vi "Create New Bucket.vi"() -> ()   [LabVIEW 2015]
doc: "Demonstrates the use of the <b>Create Bucket</b> VI in the LabVIEW Interface for Amazon S3 toolkit."
uses:
  Typedefs/AMZ_S3_LocationConstraint.ctl
  Typedefs/AMZ_S3_AWS Credentials.ctl
  Typedefs/AMZ_S3_API_PUT Bucket Request Parameters.ctl
  Typedefs/AMZ_S3_ACL.ctl
  LV Interface for Amazon S3.lvlib
panel:
  in  "Secret Key":string
  in  "Access Key":string
  in  "Bucket Name":string
  in  "Region":T1
  # "Overview: Demonstrates how to create a new Amazon S3 bucket.\nRequirements: LabVIEW Interface for Amazon S3 toolkit and a registered Amazon AWS account\nInstructions:\n1. Specify the Access Key and Secret Key for your AWS account. You can create an account at http://aws.amazon.com.\n2. Specify a Region and Bucket Name for the bucket you want to create. Note that the bucket name must be globally unique.\n3. Run the VI. Verify in the Amazon S3 console that the specified bucket was created."
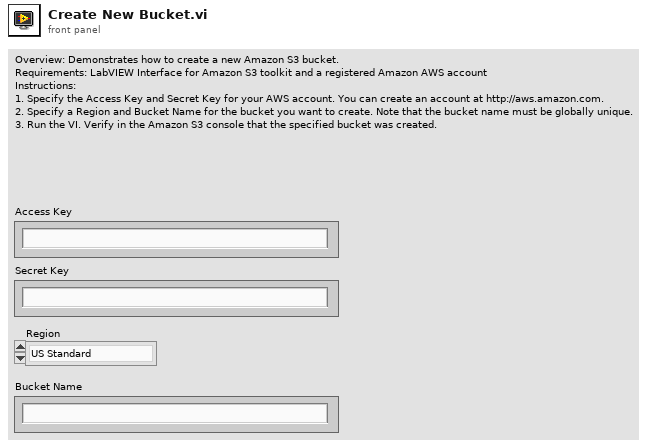
[diagram p1: front panel]
types:
  T1 = typedef "LV Interface for Amazon S3.lvlib/AMZ_S3_LocationConstraint.ctl" = enum16{"US Standard", "us-east-2", "us-west-1", "us-west-2", "ap-northeast-1", "ap-northeast-2", "ap-southeast-1", "ap-southeast-2", "ca-central-1", "eu-central-1", "eu-west-1", "eu-west-2", "sa-east-1"}
  T2 = typedef "LV Interface for Amazon S3.lvlib/AMZ_S3_AWS Credentials.ctl" = cluster{"Access Key":string, "Secret Key":string}
  T3 = typedef "LV Interface for Amazon S3.lvlib/AMZ_S3_API_PUT Bucket Request Parameters.ctl" = cluster{"ACL":T4, "Region":T1}
  T4 = typedef "LV Interface for Amazon S3.lvlib/AMZ_S3_ACL.ctl" = enum16{"private", "public-read", "public-read-write", "aws-exec-read", "authenticated-read", "bucket-owner-read", "bucket-owner-full-control"}
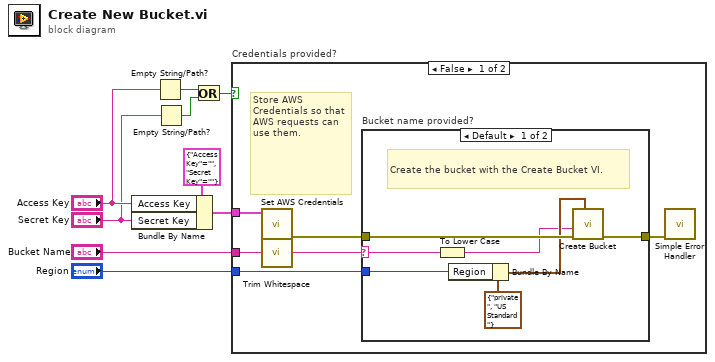
[diagram p0: block diagram]
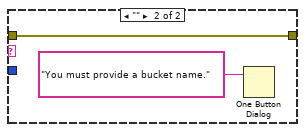
[diagram p2: hidden frame]
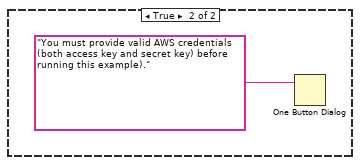
[diagram p3: hidden frame]
diagram:
  n1 = Bundle By Name(cluster=T2 {"Access Key"="", "Secret Key"=""} ("AWS Credentials in"), "Access Key"="Access Key", "Secret Key"="Secret Key") -> (w8:T2)
  n2 = Empty String/Path?(string/path="Access Key") -> (empty?=w7:bool)
  n3 = Empty String/Path?(string/path="Secret Key") -> (empty?=w5:bool)
  n4 = Or(x=w7, y=w5) -> (x .or. y?=w6:bool)
  n5 = case "Credentials provided?" shown="False" w6 {
    tunnel: w8 -> [w15 _]
    tunnel: "Bucket Name" -> [w12 _]
    tunnel: "Region" -> [w10 _]
    frame False {
      # "Store AWS Credentials so that AWS requests can use them."
      n6 = call "Set AWS Credentials.vi"("AWS Credentials in"=w15) -> ("error out"=w14:errorcluster)  [unwired: 10 in]
      n7 = call <vilib>:"Trim Whitespace.vi"("string"=w12) -> ("trimmed string"=w11:string)  [unwired: 1 in]
      n8 = case "Bucket name provided?" shown="Default" w11 {
        selector: w11 -> [w20 _]
        tunnel: w14 -> [w21 w24]
        tunnel: [w18 w24] -> w13
        tunnel: w10 -> [w17 _]
        frame Default {
          # "Create the bucket with the Create Bucket VI."
          n9 = To Lower Case(string=w20) -> (all lower case string=w16:string)
          n10 = Bundle By Name(cluster=T3 {"ACL"=enum."private", "Region"=enum."US Standard"} ("Request parameters"), "Region"=w17) -> (w19:T3)
          n11 = call "Create Bucket.vi"("Request parameters"=w19, "error in (no error)"=w21, "Bucket"=w16) -> ("error out"=w18:errorcluster)  [unwired: 8 in]
        }
        frame "" {
          n12 = One Button Dialog(message="You must provide a bucket name.") -> ()  [unwired: 1 in, 1 out]
        }
      }
      n13 = call <vilib>:"Simple Error Handler.vi"("error in (no error)"=w13) -> ()  [unwired: 4 in, 5 out]
    }
    frame True {
      n14 = One Button Dialog(message="You must provide valid AWS credentials (both access key and secret key) before running this example).") -> ()  [unwired: 1 in, 1 out]
    }
  }
